vi "HelloWorld.vi"() -> ()   [LabVIEW 2018]
panel:
  out "error out":errorcluster
  in  "Name":string="World"
  out "response":string
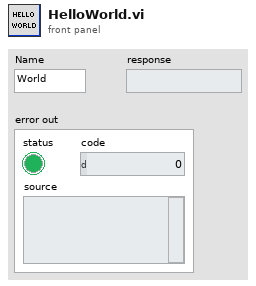
[diagram p1: front panel]
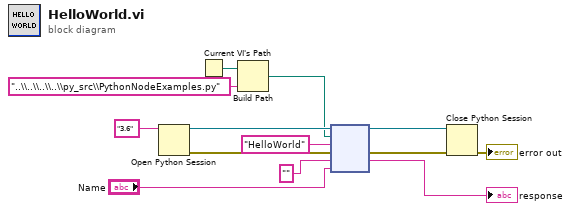
[diagram p0: block diagram]
diagram:
  n1 = Open Python Session(python version="3.6" ("Python version")) -> (session out=w13:refnum<k35>, error out=w3:errorcluster)  [unwired: 2 in]
  n2 = Current VI's Path() -> (path=w6:path)
  n3 = Build Path(base path=w6, name or relative path="..\\..\\..\\..\\py_src\\PythonNodeExamples.py") -> (appended path=w4:path)
  n4 = node(w13, w4, "HelloWorld" ("function name"), w3, "", "Name") -> (w12:refnum<k35>, w2:errorcluster, →"response":string)  [unwired: 1 in, 2 out]
  n5 = Close Python Session(session in=w12, error in=w2) -> (11:→"error out":errorcluster)
